vi "Control - EGR.vi"(8 "Control Inputs":T1={"Engine Speed [RPM]"=0.0, "Engine Status"=enum."STALLED", "Load Control \nMode"=enum."High-Idle Governor", "dt(s)"=0.0, "Number of Cylinders"=0, "Engine Displacement [cc]"=0.0, "StoichAFR"=0.0, "Q.LHV Fuel [kJ/kg]"=0.0, "BattV PSU [V]"=0.0, "12V PSU [V]"=0.0, "5V PSU [V]"=0.0, "Pedal Position [%]"=0.0, "Oil Pressure [kPa]"=0.0, "Oil Temp [C]"=0.0, "Oil Level [%]"=0.0, "Engine Coolant Temp (ECT) [C]"=0.0, "Engine Coolant Pressure [kPa]"=0.0, "Rail Pressure [bar]"=0.0, "Fuel Pressure [kPa]"=0.0, "Fuel Temp [C]"=0.0, "Vacuum Pressure [kPa]"=0.0, "Throttle Position [%]"=0.0, "Cam1 Advance [CAD]"=0.0, "Cam2 Advance [CAD]"=0.0, "Cam3 Advance [CAD]"=0.0, "Cam4 Advance [CAD]"=0.0, "CA50 Control Output [CAD]"=[], "CA50 Control Output Valid"=[], "Intake Air Temp (IAT) [C]"=0.0, "Barometric Air Pressure [kPa]"=0.0, "Intake Air Rel. Humidity [%]"=0.0, "Mass Air Flow (MAF) [kg/hr]"=0.0, "Turbo Inlet Air Pressure [kPa]"=0.0, "Turbo Inlet Air Temp [C]"=0.0, "Turbo Outlet Air Pressure [kPa]"=0.0, "Turbo Outlet Air Temp [C]"=0.0, "CAC Outlet Pressure [kPa]"=0.0, "CAC Outlet Temp [C]"=0.0, "Intake Manifold Pressure (MAP) [kPa]"=0.0, "Intake Manifold Temp (MAT) [C]"=0.0, "Exhaust Manifold Pressure [kPa]"=0.0, "Exhaust Manifold Temp [C]"=0.0, "HighP EGR Cooler Outlet Pressure [kPa]"=0.0, "HighP EGR Cooler Outlet Temp [C]"=0.0, "HighP EGR Differential Pressure [kPa]"=0.0, "HighP EGR Valve Position [%]"=0.0, "Turbo Outlet Exhaust Pressure [kPa]"=0.0, "Turbo Outlet Exhaust Temp [C]"=0.0, "VGT Position 1 [%]"=0.0, "VGT Position 2 [%]"=0.0, "Turbo Speed 1 [RPM]"=0.0, "Turbo Speed 2 [RPM]"=0.0, "LowP EGR Differential Pressure [kPa]"=0.0, "LowP EGR Valve Position [%]"=0.0, "UEGO1Lambda"=0.0, "UEGO1_Hot"=FALSE, "UEGO2Lambda"=0.0, "UEGO2_Hot"=FALSE, "Knock Intensity"=[], "Knock"=[]} {"Knock Intensity" format="%.2f"; "CA50 Control Output [CAD]" format="%.2f"; "Exhaust Manifold Temp [C]" format="%#_6f"; "UEGO2Lambda" format="%.2f"; "Intake Manifold Temp (MAT) [C]" format="%#_6f"; "UEGO1Lambda" format="%.2f"}, 10 "MEP Desired [bar]":sgl, 11 "EGR Mass [mg/cyc]":sgl) -> (1 "Low-Pressure EGR Position [%Open]":sgl, 3 "High-Pressure EGR Position [%Open]":sgl)   [LabVIEW 2015, in "ECS-RT.lvlib"]
uses:
  ECS-RT.lvlib
  Typedefs/Control Inputs/Control Inputs.ctl
  Typedefs/EPT/Engine Status.ctl
  Typedefs/MISC/Load Control Mode.ctl
  ECS-Shared.lvlib
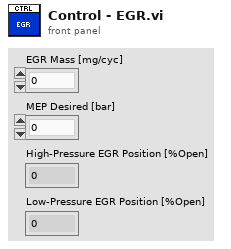
[diagram p1: front panel]
types:
  T1 = typedef "ECS-Shared.lvlib/Control Inputs.ctl" = cluster{"Engine Speed [RPM]":sgl, "Engine Status":T2, "Load Control \nMode":T3, "dt(s)":sgl, "Number of Cylinders":u8, "Engine Displacement [cc]":sgl, "StoichAFR":sgl, "Q.LHV Fuel [kJ/kg]":sgl, "BattV PSU [V]":sgl, "12V PSU [V]":sgl, "5V PSU [V]":sgl, "Pedal Position [%]":sgl, "Oil Pressure [kPa]":sgl, "Oil Temp [C]":sgl, "Oil Level [%]":sgl, "Engine Coolant Temp (ECT) [C]":sgl, "Engine Coolant Pressure [kPa]":sgl, "Rail Pressure [bar]":sgl, "Fuel Pressure [kPa]":sgl, "Fuel Temp [C]":sgl, "Vacuum Pressure [kPa]":sgl, "Throttle Position [%]":sgl, "Cam1 Advance [CAD]":sgl, "Cam2 Advance [CAD]":sgl, "Cam3 Advance [CAD]":sgl, "Cam4 Advance [CAD]":sgl, "CA50 Control Output [CAD]":sgl[], "CA50 Control Output Valid":bool[], "Intake Air Temp (IAT) [C]":sgl, "Barometric Air Pressure [kPa]":sgl, "Intake Air Rel. Humidity [%]":sgl, "Mass Air Flow (MAF) [kg/hr]":sgl, "Turbo Inlet Air Pressure [kPa]":sgl, "Turbo Inlet Air Temp [C]":sgl, "Turbo Outlet Air Pressure [kPa]":sgl, "Turbo Outlet Air Temp [C]":sgl, "CAC Outlet Pressure [kPa]":sgl, "CAC Outlet Temp [C]":sgl, "Intake Manifold Pressure (MAP) [kPa]":sgl, "Intake Manifold Temp (MAT) [C]":sgl, "Exhaust Manifold Pressure [kPa]":sgl, "Exhaust Manifold Temp [C]":sgl, "HighP EGR Cooler Outlet Pressure [kPa]":sgl, "HighP EGR Cooler Outlet Temp [C]":sgl, "HighP EGR Differential Pressure [kPa]":sgl, "HighP EGR Valve Position [%]":sgl, "Turbo Outlet Exhaust Pressure [kPa]":sgl, "Turbo Outlet Exhaust Temp [C]":sgl, "VGT Position 1 [%]":sgl, "VGT Position 2 [%]":sgl, "Turbo Speed 1 [RPM]":sgl, "Turbo Speed 2 [RPM]":sgl, "LowP EGR Differential Pressure [kPa]":sgl, "LowP EGR Valve Position [%]":sgl, "UEGO1Lambda":sgl, "UEGO1_Hot":bool, "UEGO2Lambda":sgl, "UEGO2_Hot":bool, "Knock Intensity":sgl[], "Knock":bool[]}
  T2 = typedef "ECS-Shared.lvlib/Engine Status.ctl" = enum16{"OFF", "STALLED", "CRANKING", "RUNNING", "ACCEL", "DECEL", "SAFE"}
  T3 = typedef "ECS-Shared.lvlib/Load Control Mode.ctl" = enum16{"No Governor", "Low-Idle Governor", "High-Idle Governor"}
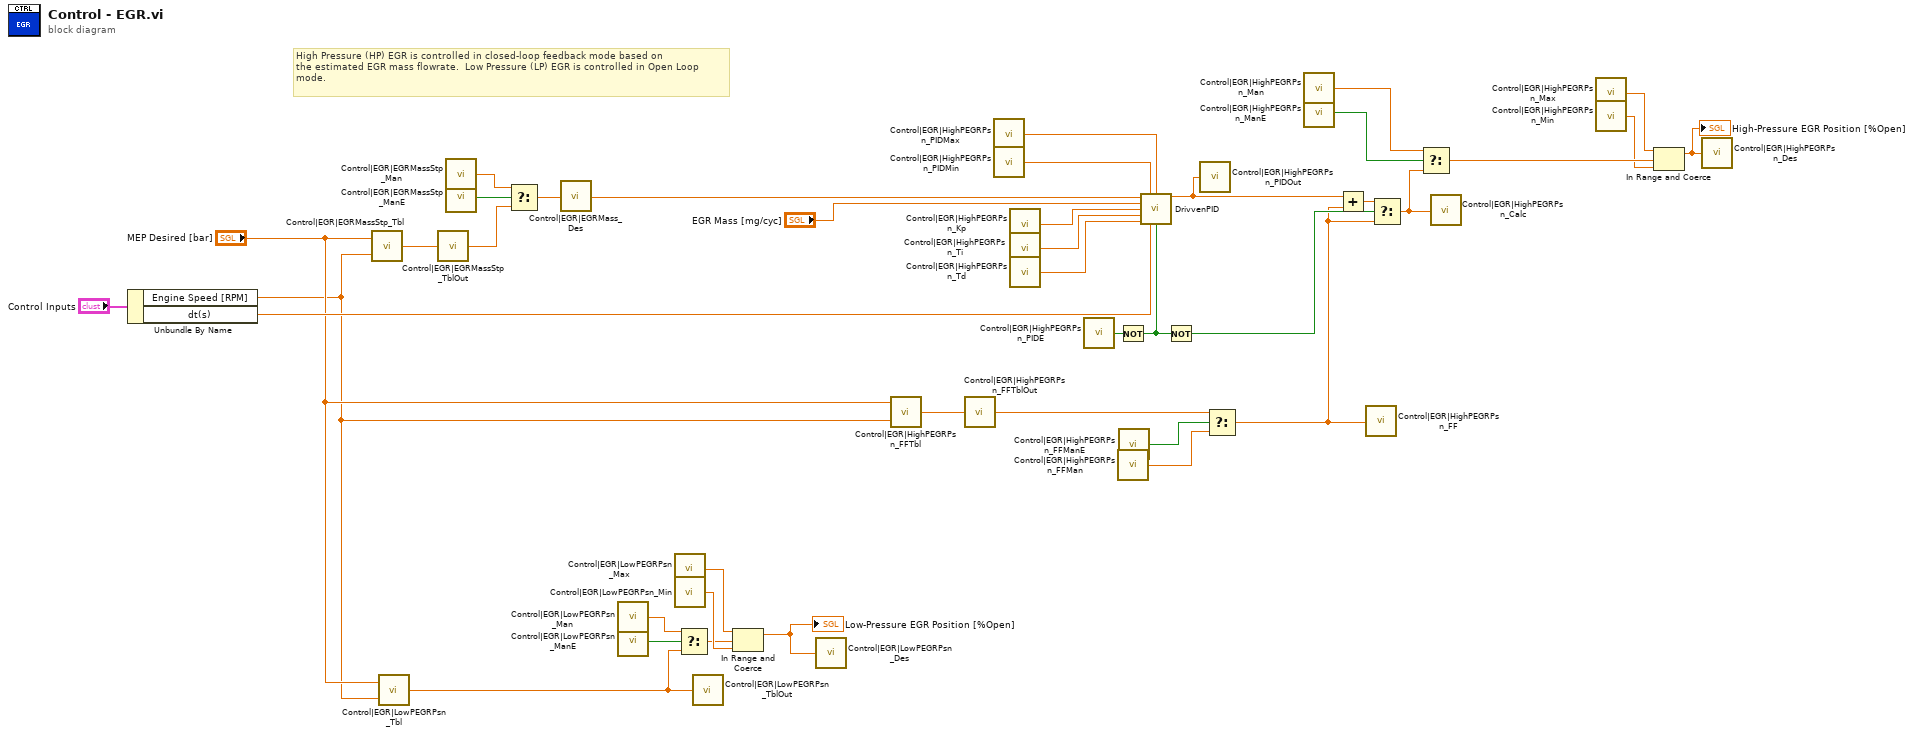
[diagram p0: block diagram]
diagram:
  # "High Pressure (HP) EGR is controlled in closed-loop feedback mode based on\nthe estimated EGR mass flowrate.  Low Pressure (LP) EGR is controlled in Open Loop mode."
  n1 = Unbundle By Name("Control Inputs") -> ("Engine Speed [RPM]"=w3:sgl, "dt(s)"=w28:sgl)
  n2 = call "Control|EGR|EGRMassStp_Tbl"("Y Index"=w3, "X Index"="MEP Desired [bar]") -> ("Z"=w18:sgl)
  n3 = call "Control|EGR|LowPEGRPsn_Tbl"("Y Index"=w3, "X Index"="MEP Desired [bar]") -> ("Z"=w24:sgl)
  n4 = call "Control|EGR|EGRMassStp_TblOut"("Value"=w18) -> ()
  n5 = call "Control|EGR|EGRMassStp_Man"() -> ("Value"=w20:sgl)
  n6 = call "Control|EGR|EGRMassStp_ManE"() -> ("Value"=w19:bool)
  n7 = Select(t=w20, s=w19, f=w18) -> (s? t:f=w17:sgl)
  n8 = call "Control|EGR|EGRMass_Des"("Value"=w17) -> ()
  n9 = call "Control|EGR|LowPEGRPsn_Man"() -> ("Value"=w25:sgl)
  n10 = call "Control|EGR|LowPEGRPsn_ManE"() -> ("Value"=w26:bool)
  n11 = call "Control|EGR|LowPEGRPsn_Max"() -> ("Value"=w11:sgl)
  n12 = call "Control|EGR|LowPEGRPsn_Min"() -> ("Value"=w10:sgl)
  n13 = Select(t=w25, s=w26, f=w24) -> (s? t:f=w9:sgl)
  n14 = call "Control|EGR|LowPEGRPsn_TblOut"("Value"=w24) -> ()
  n15 = In Range and Coerce(upper limit=w11, x=w9, lower limit=w10) -> (coerced(x)=w8:sgl)  [unwired: 1 out]
  "Low-Pressure EGR Position [%Open]" <- w8
  n16 = call "Control|EGR|LowPEGRPsn_Des"("Value"=w8) -> ()
  n17 = call "Control|EGR|HighPEGRPsn_FFTbl"("Y Index"=w3, "X Index"="MEP Desired [bar]") -> ("Z"=w2:sgl)
  n18 = call "Control|EGR|HighPEGRPsn_FFTblOut"("Value"=w2) -> ()
  n19 = call "Control|EGR|HighPEGRPsn_PIDMax"() -> ("Value"=w36:sgl)
  n20 = call "Control|EGR|HighPEGRPsn_PIDMin"() -> ("Value"=w37:sgl)
  n21 = call "Control|EGR|HighPEGRPsn_Kp"() -> ("Value"=w32:sgl)
  n22 = call "Control|EGR|HighPEGRPsn_Ti"() -> ("Value"=w33:sgl)
  n23 = call "Control|EGR|HighPEGRPsn_Td"() -> ("Value"=w34:sgl)
  n24 = call "Control|EGR|HighPEGRPsn_PIDE"() -> ("Value"=w35:bool)
  n25 = Not(x=w35) -> (.not. x?=w23:bool)
  n26 = call "Control|EGR|HighPEGRPsn_FFMan"() -> ("Value"=w5:sgl)
  n27 = call "Control|EGR|HighPEGRPsn_FFManE"() -> ("Value"=w27:bool)
  n28 = call <vilib>:"DrivvenPID.vi"("Setpoint"=w17, "OutputLow"=w37, "OutputHigh"=w36, "ProcessVariable"="EGR Mass [mg/cyc]", "ProportionalGain (Kc)"=w32, "IntegralTime (Ti, min)"=w33, "DerivativeTime (Td, min)"=w34, "dt (s)"=w28, "Reinitialize? (F)"=w23) -> ("Output"=w1:sgl)  [unwired: 6 out]
  n29 = Not(x=w23) -> (.not. x?=w22:bool)
  n30 = call "Control|EGR|HighPEGRPsn_PIDOut"("Value"=w1) -> ()
  n31 = Select(t=w2, s=w27, f=w5) -> (s? t:f=w6:sgl)
  n32 = call "Control|EGR|HighPEGRPsn_Man"() -> ("Value"=w31:sgl)
  n33 = call "Control|EGR|HighPEGRPsn_ManE"() -> ("Value"=w30:bool)
  n34 = Add(x=w1, y=w6) -> (x+y=w7:sgl)
  n35 = call "Control|EGR|HighPEGRPsn_FF"("Value"=w6) -> ()
  n36 = Select(t=w7, s=w22, f=w6) -> (s? t:f=w16:sgl)
  n37 = Select(t=w31, s=w30, f=w16) -> (s? t:f=w15:sgl)
  n38 = call "Control|EGR|HighPEGRPsn_Calc"("Value"=w16) -> ()
  n39 = call "Control|EGR|HighPEGRPsn_Max"() -> ("Value"=w13:sgl)
  n40 = call "Control|EGR|HighPEGRPsn_Min"() -> ("Value"=w14:sgl)
  n41 = In Range and Coerce(upper limit=w13, x=w15, lower limit=w14) -> (coerced(x)=w12:sgl)  [unwired: 1 out]
  "High-Pressure EGR Position [%Open]" <- w12
  n42 = call "Control|EGR|HighPEGRPsn_Des"("Value"=w12) -> ()
